vi "open camera quick settings.vi"(8 "error in (no error)":errorcluster, 9 "Open?":bool, 10 "SubPanel Ref":refnum<vi>, 11 "IMAQdx Actor in":refnum<class "IMAQdx Actor.lvclass">) -> (0 "error out":errorcluster, 3 "IMAQdx Actor out":refnum<class "IMAQdx Actor.lvclass">)   [LabVIEW 2014, in "IMAQdx Actor.lvlib" / "IMAQdx Actor.lvclass"]
uses:
  IMAQdx Actor.lvclass
  IMAQdx Actor.lvclass/IMAQdx Actor.ctl
  Camera Quick Settings Panel/Camera Settings Dialog/Camera Quick Settings Panel.lvclass
  Camera Quick Settings Panel/Camera Settings Dialog/Camera Quick Settings Panel.lvclass/Camera Quick Settings Panel.ctl
  Shared Code/Viewable Actor/ViewableActor Messages/Insert Into SubPanel Msg/Insert Into SubPanel Msg.lvclass/Insert Into SubPanel Msg.ctl
  <vilib>/ActorFramework/Message Enqueuer/Message Enqueuer.lvclass/Message Enqueuer.ctl
  Camera Quick Settings Panel/Camera Settings Dialog/Write Exposure Time abs Attr.vi
  Camera Quick Settings Panel/Camera Settings Dialog/Write Trigger Mode Attr.vi
  Camera Quick Settings Panel/Camera Settings Dialog/Write IMAQdx Session.vi
  <vilib>/ActorFramework/Message Enqueuer/Enqueue.vi
  <vilib>/ActorFramework/Message Priority Queue/Priority Enqueue.vi
  <vilib>/ActorFramework/Message Enqueuer/Message Enqueuer.lvclass
  Shared Code/Viewable Actor/ViewableActor Messages/Insert Into SubPanel Msg/Insert Into SubPanel Msg.lvclass
  Shared Code/Viewable Actor/ViewableActor Messages/Open Front Panel Msg/Open Front Panel Msg.lvclass
  <vilib>/ActorFramework/Actor/Actor.lvclass
  <resource>/objmgr/imaqdx.rc
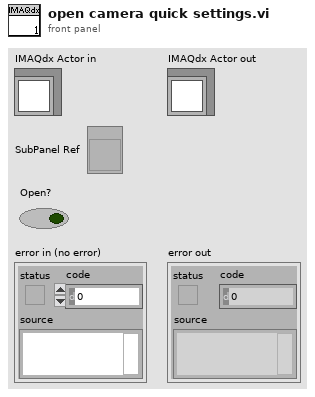
[diagram p1: front panel]
types:
  T1 = typedef "IMAQdx.ctl" = refnum<k21>
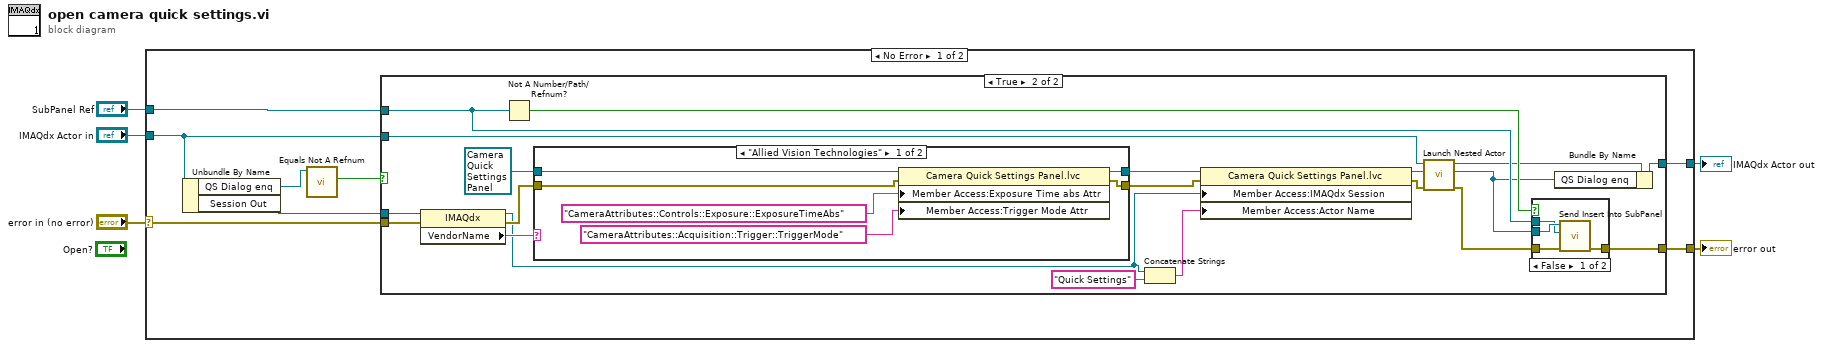
[diagram p0: block diagram]
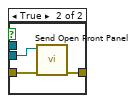
[diagram p4: hidden frame]
diagram:
  n1 = case shown="No Error" "error in (no error)" {
    selector: "error in (no error)" -> [w9 w52]
    tunnel: [w11 w52] -> w4
    tunnel: [w8 w51] -> w2
    tunnel: "IMAQdx Actor in" -> [w12 w51]
    tunnel: "SubPanel Ref" -> [w13 _]
    frame No Error {
      n2 = Unbundle By Name(w12) -> ("QS Dialog enq"=w6:refnum<class "Message Enqueuer.lvclass">, "Session Out"=w10:T1)
      n3 = call <vilib>:"Equals Not A Refnum.vi"("Message Enqueuer"=w6) -> ("Not a refnum?"=w7:bool)  [unwired: 10 in]
      n4 = case shown="True" w7 {
        tunnel: w13 -> [_ w34]
        tunnel: w12 -> [w15 w31]
        tunnel: [w14 w29] -> w11
        tunnel: w10 -> [_ w28]
        tunnel: w9 -> [w14 w22]
        tunnel: [w15 w17] -> w8
        frame False {
        }
        frame True {
          n5 = property class="IMAQdx"(reference=w28, error in=w22) -> (reference out=w19:T1, error out=w24:errorcluster, "VendorName"=w27:string)
          n6 = Not A Number/Path/Refnum?(number/path/refnum=w34) -> (NaN/Path/Refnum?=w35:bool)
          n7 = case shown="\"Allied Vision Technologies\"" w27 {
            tunnel: [w40 w43] -> w26
            tunnel: refnum<class "Camera Quick Settings Panel.lvclass"> refnum ("Camera Quick Settings Panel.lvlib:Camera Settings Dialog.lvclass") -> [w41 w43]
            tunnel: w24 -> [w39 w42]
            tunnel: [w38 w42] -> w23
            frame "Allied Vision Technologies" {
              n8 = property class="Camera Quick Settings Panel.lvc"(reference=w41, error in=w39, "Member Access:Exposure Time abs Attr"="CameraAttributes::Controls::Exposure::ExposureTimeAbs" ("Exposure Time abs Attr"), "Member Access:Trigger Mode Attr"="CameraAttributes::Acquisition::Trigger::TriggerMode" ("Trigger Mode Attr")) -> (reference out=w40:refnum<class "Camera Quick Settings Panel.lvclass">, error out=w38:errorcluster)
            }
            frame "Basler", Default {
            }
          }
          n9 = Concatenate Strings(w19, "Quick Settings" ("string")) -> (w18:string)
          n10 = property class="Camera Quick Settings Panel.lvc"(reference=w26, error in=w23, "Member Access:IMAQdx Session"=w19, "Member Access:Actor Name"=w18) -> (reference out=w32:refnum<class "Camera Quick Settings Panel.lvclass">, error out=w21:errorcluster)
          n11 = call <vilib>:"Launch Nested Actor.vi"("error in (no error)"=w21, "Nested Actor"=w32, "Caller Actor in"=w31) -> ("error out"=w30:errorcluster, "Nested Actor's Enqueuer"=w16:refnum<class "Message Enqueuer.lvclass">, "Caller Actor out"=w33:refnum<class "IMAQdx Actor.lvclass">)  [unwired: 6 in]
          n12 = case shown="False" w35 {
            tunnel: w16 -> [w47 w50]
            tunnel: w30 -> [w46 w49]
            tunnel: [w45 w48] -> w29
            tunnel: w34 -> [w44 _]
            frame False {
              n13 = call "Send Insert Into SubPanel.vi"("error in (no error)"=w46, "SubPanel Ref"=w44, "Message Enqueuer"=w47) -> ("error out"=w45:errorcluster)  [unwired: 7 in, 1 out]
            }
            frame True {
              n14 = call "Send Open Front Panel.vi"("error in (no error)"=w49, "Message Enqueuer"=w50) -> ("error out"=w48:errorcluster)  [unwired: 8 in, 1 out]
            }
          }
          n15 = Bundle By Name(cluster=w33, "QS Dialog enq"=w16) -> (w17:refnum<class "IMAQdx Actor.lvclass">)
        }
      }
    }
    frame Error {
    }
  }
  "error out" <- w4
  "IMAQdx Actor out" <- w2
